vi "Automatic Extruder LabVIEW Program.vi"() -> ()   [LabVIEW 2022 SP3]
doc: "This VI allows to perform a single run pumping mode : the pump run continuously until the user decide to stop, reverse or pause it."
uses:
  <vilib>/Utility/error.llb/DialogType.ctl
  <vilib>/ptbypt/NI_PtbyPt.lvlib
panel:
  out "?":string
  out "Tank 4":dbl(slide) scale=0.0..1.0
  out "Tank 3":dbl(slide) scale=0.0..1000.0
  in  "Volume":string(combo)
  out "?":string
  out "Firmware Version :  2":string
  out "Extrusions Completed":i32
  out "Firmware Version :":string
  in  "Baud Rate (19200)":u32(ring)=19200 items=["19200"=19200, "9600"=9600, "2400"=2400, "1200"=1200, "300"=300]
  in  "Extrusions To Preform":i32
  in  "Master Pump Address":i32 format="%0#.0f"
  in  "Secondary Pump Resource":refnum<visa-resource-name>="COM4"
  in  "Master Pump VISA Resource":refnum<visa-resource-name>="COM3"
  in  "Secondary Pump Address":i32=1 format="%0#.0f"
  out "Tank 2":dbl(slide) scale=0.0..1000.0
  out "x+y":i32
  out "Tank":dbl(slide) scale=0.0..1.0
  in  "PAUSE 2":bool
  in  "PAUSE":bool
  in  "RUN":bool
  in  "STOP":bool
  in  "Audible Alarms":bool=TRUE
  in  "Flow rate":dbl=0.5 format="%.3f"
  in  "Units":i32(ring) items=["microlitters per minute (µL/min)", "microlitters per hour (µL/hr)", "milliliters per minute (mL/min)", "milliliters per hour (mL/hr)"]
  in  "Initial Direction":u16(ring) items=["Infuse", "Withdraw"]
  in  "Syringe Inside Diameter \nIf diameter is greater than 14.00 mm : Volume units are mL\nIf diameter is less than 14.00 mm : Volume units are µL":dbl=20.0 min=1.0 max=50.0 step=1.0
  out "Status":T1
  # "Configuration Settings"
  # "Master Pump Status"
  # "Volume"
  # "mm"
  # "Pump Control"
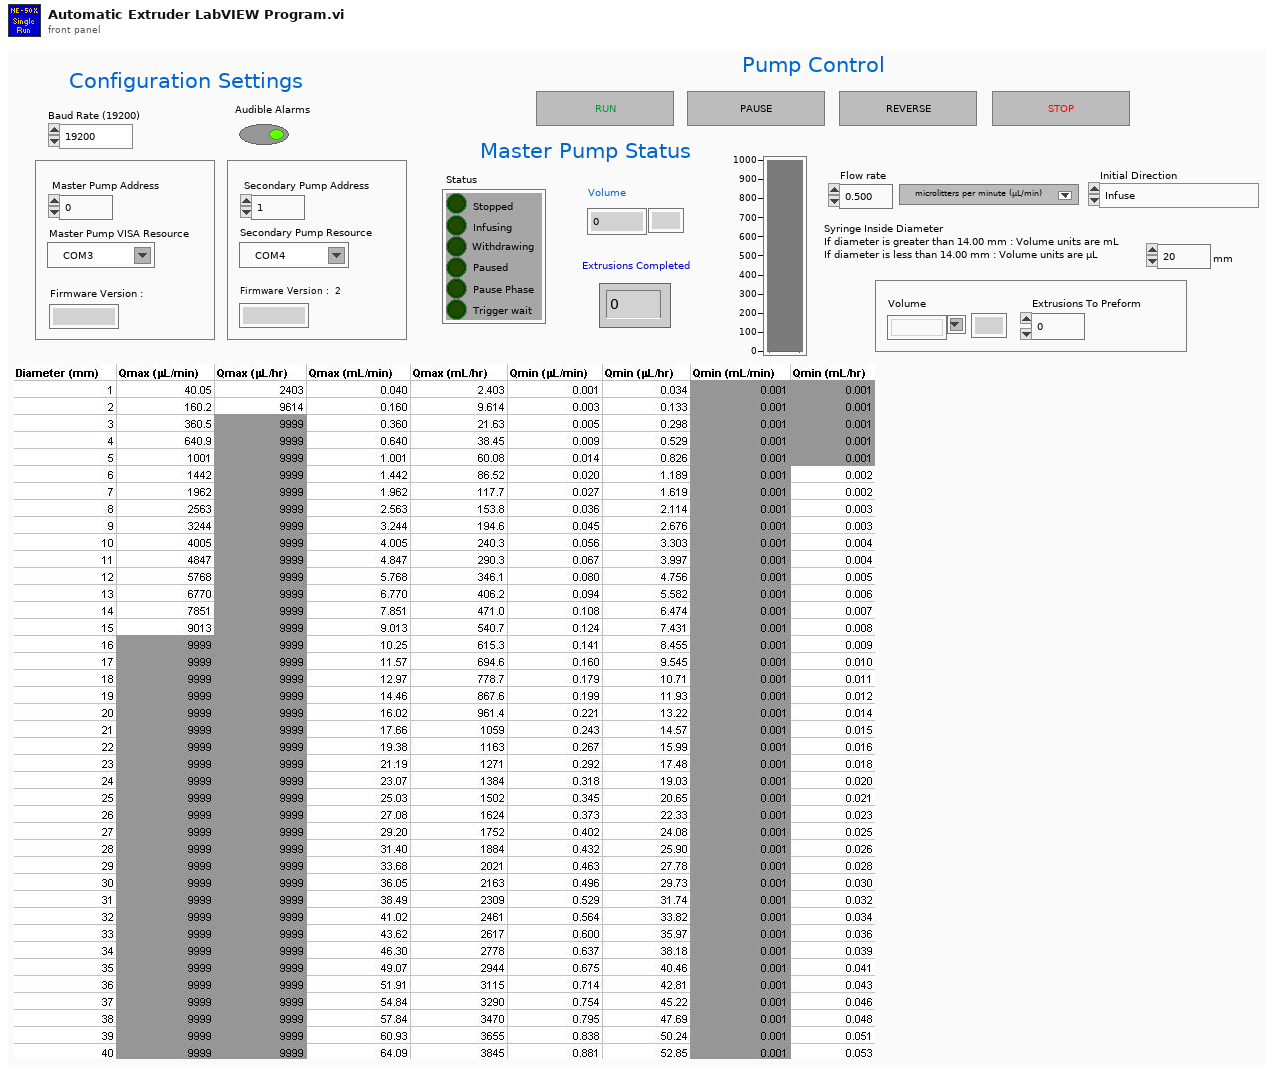
[diagram p1: front panel]
types:
  T1 = cluster{"Stopped":bool, "Infusing":bool, "Withdrawing":bool, "Paused":bool, "Pause Phase":bool, "Trigger wait":bool}
  T2 = typedef "DialogType.ctl" = u16
  T3 = cluster{"0=off\n1=on":u16, "Numbers of beeps\n0=continuously":dbl}
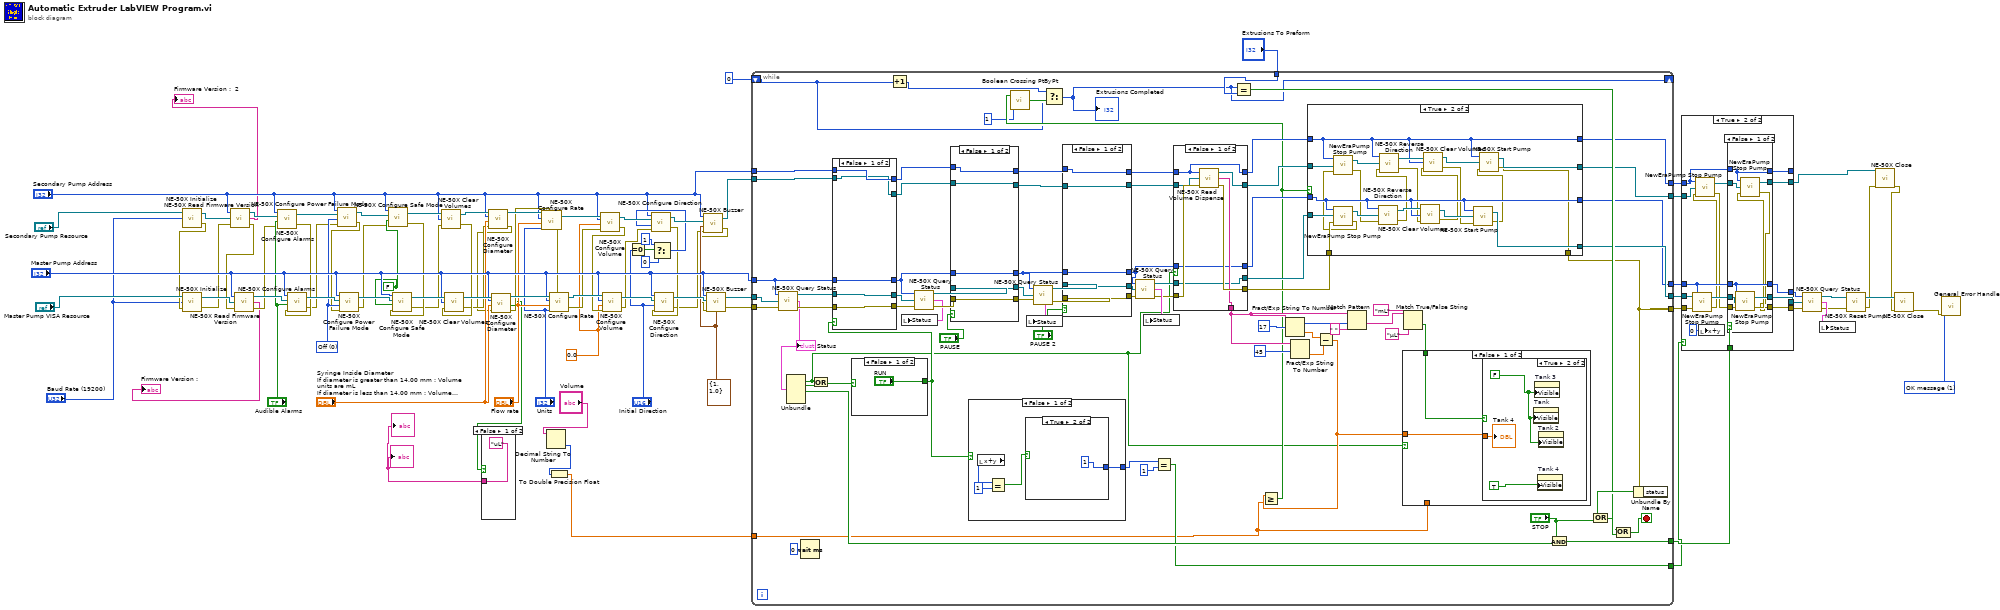
[diagram p0: block diagram]
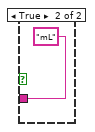
[diagram p2: hidden frame]
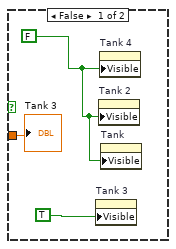
[diagram p5: hidden frame]
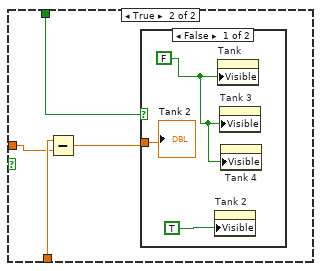
[diagram p6: hidden frame]
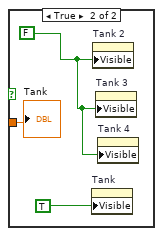
[diagram p7: hidden frame]
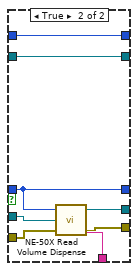
[diagram p8: hidden frame]
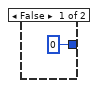
[diagram p10: hidden frame]
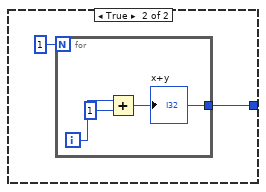
[diagram p11: hidden frame]
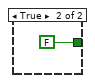
[diagram p12: hidden frame]
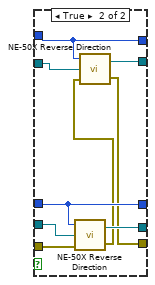
[diagram p13: hidden frame]
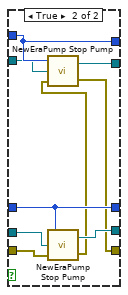
[diagram p14: hidden frame]
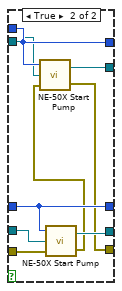
[diagram p15: hidden frame]
diagram:
  w8 = 0.0
  w70 = T2 1 items=["no dialog", "OK message", "continue or stop message", "OK message + warnings", "continue/stop + warnings"] ("type of dialog (OK msg:1)")
  w52 = FALSE ("0 = Basic")
  w51 = u16 0 items=["Off", "On"] ("0 = Disabled")
  w47 = T3 {"0=off\n1=on"=1, "Numbers of beeps\n0=continuously"=1.0} ("Buzzer")
  n1 = call <instrlib>:"NE-50X Initialize.vi"("Baud Rate (19200)"="Baud Rate (19200)", "VISA resource name"="Secondary Pump Resource") -> ("error out"=w40:errorcluster, "VISA resource name out"=w62:refnum<visa-resource-name>)  [unwired: 1 in]
  n2 = call <instrlib>:"NE-50X Initialize.vi"("error in (no error)"=w40, "Baud Rate (19200)"="Baud Rate (19200)", "VISA resource name"="Master Pump VISA Resource") -> ("error out"=w39:errorcluster, "VISA resource name out"=w78:refnum<visa-resource-name>)
  n3 = call <instrlib>:"NE-50X Read Firmware Version.vi"("error in (no error)"=w39, "VISA resource name"=w62, "Address (0)"="Secondary Pump Address") -> ("error out"=w38:errorcluster, "Version"=→"Firmware Version :  2":string, "VISA resource name out"=w61:refnum<visa-resource-name>)
  n4 = call <instrlib>:"NE-50X Read Firmware Version.vi"("error in (no error)"=w38, "VISA resource name"=w78, "Address (0)"="Master Pump Address") -> ("error out"=w37:errorcluster, "Version"=→"Firmware Version :":string, "VISA resource name out"=w79:refnum<visa-resource-name>)
  n5 = call <instrlib>:"NE-50X Configure Alarms.vi"("error in (no error)"=w37, "Audible Alarms"="Audible Alarms", "VISA resource name"=w61, "Address (0)"="Secondary Pump Address") -> ("error out"=w36:errorcluster, "VISA resource name out"=w60:refnum<visa-resource-name>)
  n6 = call <instrlib>:"NE-50X Configure Alarms.vi"("error in (no error)"=w36, "Audible Alarms"="Audible Alarms", "VISA resource name"=w79, "Address (0)"="Master Pump Address") -> ("error out"=w35:errorcluster, "VISA resource name out"=w80:refnum<visa-resource-name>)
  n7 = call <instrlib>:"NE-50X Configure Power Failure Mode.vi"("error in (no error)"=w35, "Power Failure Mode"=w51, "VISA resource name"=w60, "Address (0)"="Secondary Pump Address") -> ("error out"=w34:errorcluster, "VISA resource name out"=w59:refnum<visa-resource-name>)
  n8 = call <instrlib>:"NE-50X Configure Power Failure Mode.vi"("error in (no error)"=w34, "Power Failure Mode"=w51, "VISA resource name"=w80, "Address (0)"="Master Pump Address") -> ("error out"=w33:errorcluster, "VISA resource name out"=w81:refnum<visa-resource-name>)
  n9 = call <instrlib>:"NE-50X Configure Safe Mode.vi"("error in (no error)"=w33, "Safe Mode"=w52, "VISA resource name"=w59, "Address (0)"="Secondary Pump Address") -> ("error out"=w32:errorcluster, "VISA resource name out"=w58:refnum<visa-resource-name>)
  n10 = call <instrlib>:"NE-50X Configure Safe Mode.vi"("error in (no error)"=w32, "Safe Mode"=w52, "VISA resource name"=w81, "Address (0)"="Master Pump Address") -> ("error out"=w31:errorcluster, "VISA resource name out"=w69:refnum<visa-resource-name>)
  n11 = call <instrlib>:"NE-50X Clear Volumes.vi"("error in (no error)"=w31, "Address (0)"="Secondary Pump Address", "VISA resource name"=w58) -> ("error out"=w30:errorcluster, "VISA resource name out"=w57:refnum<visa-resource-name>)
  n12 = call <instrlib>:"NE-50X Clear Volumes.vi"("error in (no error)"=w30, "Address (0)"="Master Pump Address", "VISA resource name"=w69) -> ("error out"=w29:errorcluster, "VISA resource name out"=w66:refnum<visa-resource-name>)
  n13 = call <instrlib>:"NE-50X Configure Diameter.vi"("error in (no error)"=w29, "Diameter (19.58 mm)"="Syringe Inside Diameter \nIf diameter is greater than 14.00 mm : Volume units are mL\nIf diameter is less than 14.00 mm : Volume units are µL", "Address (0)"="Secondary Pump Address", "VISA resource name"=w57) -> ("error out"=w28:errorcluster, "VISA resource name out"=w56:refnum<visa-resource-name>)  [unwired: 1 in, 1 out]
  n14 = call <instrlib>:"NE-50X Configure Diameter.vi"("error in (no error)"=w28, "Diameter (19.58 mm)"="Syringe Inside Diameter \nIf diameter is greater than 14.00 mm : Volume units are mL\nIf diameter is less than 14.00 mm : Volume units are µL", "Address (0)"="Master Pump Address", "VISA resource name"=w66) -> ("error out"=w27:errorcluster, "Volume units"=w10:bool, "VISA resource name out"=w67:refnum<visa-resource-name>)  [unwired: 1 in]
  n15 = case shown="False" w10 {
    tunnel: ["uL" "mL"] -> w1
    frame False {
    }
    frame True {
    }
  }
  "?" <- w1
  "?" <- w1
  n16 = call <instrlib>:"NE-50X Configure Rate.vi"("VISA resource name"=w56, "Address (0)"="Secondary Pump Address", "Flow"="Flow rate", "Units"="Units", "error in (no error)"=w27) -> ("VISA resource name out"=w55:refnum<visa-resource-name>, "error out"=w26:errorcluster)
  n17 = Decimal String To Number(string="Volume") -> (number=w6:i32)  [unwired: 2 in, 1 out]
  n18 = call <instrlib>:"NE-50X Configure Rate.vi"("VISA resource name"=w67, "Address (0)"="Master Pump Address", "Flow"="Flow rate", "Units"="Units", "error in (no error)"=w26) -> ("VISA resource name out"=w68:refnum<visa-resource-name>, "error out"=w25:errorcluster)
  n19 = To Double Precision Float(number=w6) -> (double precision float=w5:dbl)
  n20 = call <instrlib>:"NE-50X Configure Volume.vi"("error in (no error)"=w25, "Volume"=w8, "Address (0)"="Secondary Pump Address", "VISA resource name"=w55) -> ("error out"=w24:errorcluster, "VISA resource name out"=w54:refnum<visa-resource-name>)
  n21 = call <instrlib>:"NE-50X Configure Volume.vi"("error in (no error)"=w24, "Volume"=w8, "Address (0)"="Master Pump Address", "VISA resource name"=w68) -> ("error out"=w23:errorcluster, "VISA resource name out"=w82:refnum<visa-resource-name>)
  n22 = Equal To 0?(x="Initial Direction") -> (x = 0?=w45:bool)
  n23 = Select(t=u16 1, s=w45, f=u16 0) -> (s? t:f=w41:u16)
  n24 = call <instrlib>:"NE-50X Configure Direction.vi"("error in (no error)"=w23, "Direction"=w41, "VISA resource name"=w54, "Address (0)"="Secondary Pump Address") -> ("error out"=w22:errorcluster, "VISA resource name out"=w53:refnum<visa-resource-name>)
  n25 = call <instrlib>:"NE-50X Configure Direction.vi"("error in (no error)"=w22, "Direction"="Initial Direction", "VISA resource name"=w82, "Address (0)"="Master Pump Address") -> ("error out"=w21:errorcluster, "VISA resource name out"=w83:refnum<visa-resource-name>)
  n26 = call <instrlib>:"NE-50X Buzzer.vi"("error in (no error)"=w21, "Buzzer"=w47, "VISA resource name"=w53, "Address (0)"="Secondary Pump Address") -> ("error out"=w20:errorcluster, "VISA resource name out"=w18:refnum<visa-resource-name>)
  n27 = call <instrlib>:"NE-50X Buzzer.vi"("error in (no error)"=w20, "Buzzer"=w47, "VISA resource name"=w83, "Address (0)"="Master Pump Address") -> ("error out"=w86:errorcluster, "VISA resource name out"=w85:refnum<visa-resource-name>)
  n28 = while {
    tunnel: w85 -> [w149]
    tunnel: w86 -> [w170]
    tunnel: [w118] -> w77
    tunnel: [w119] -> w84
    tunnel: "Master Pump Address" -> [w148]
    tunnel: [w115] -> w76
    tunnel: [w141] -> w74
    tunnel: [w137] -> w72
    tunnel: "Secondary Pump Address" -> [w131]
    tunnel: w18 -> [w129]
    tunnel: [w117] -> w16
    tunnel: [w114] -> w17
    tunnel: w5 -> [w93]
    tunnel: "Extrusions To Preform" -> [w116]
    shift-right: [w97] -> _
    shift-left: 0 -> [w98]
    stop <- w122 stop-if-true
    n29 = call <instrlib>:"NE-50X Query Status.vi"("error in (no error)"=w170, "VISA resource name"=w149, "Address (0)"=w148) -> ("error out"=w167:errorcluster, "Status"=w161:T1, "VISA resource name out"=w168:refnum<visa-resource-name>)
    "Status" <- w161
    n30 = Unbundle(w161) -> ("Infusing"=w94:bool, "Withdrawing"=w160:bool, "Paused"=w142:bool)  [unwired: 3 out]
    n31 = Wait (ms)(milliseconds to wait=u32 0) -> ()  [unwired: 1 out]
    n32 = Or(x=w94, y=w160) -> (x .or. y?=w159:bool)
    n33 = case shown="False" w159 {
      tunnel: ["RUN" FALSE ("RUN")] -> w138
      frame False {
      }
      frame True {
      }
    }
    n34 = case shown="False" w138 {
      tunnel: w148 -> [w277 w283]
      tunnel: [w276 w286] -> w145
      tunnel: [w275 w278] -> w158
      tunnel: [w277 w283] -> w147
      tunnel: w168 -> [w276 w284]
      tunnel: w167 -> [w275 w285]
      tunnel: w131 -> [w274 w282]
      tunnel: [w274 w282] -> w130
      tunnel: w129 -> [w273 w281]
      tunnel: [w273 w280] -> w128
      frame False {
      }
      frame True {
        n35 = call <instrlib>:"NE-50X Start Pump.vi"("error in (no error)"=w285, "VISA resource name"=w284, "Address (0)"=w283) -> ("error out"=w279:errorcluster, "VISA resource name out"=w286:refnum<visa-resource-name>)
        n36 = call <instrlib>:"NE-50X Start Pump.vi"("error in (no error)"=w279, "VISA resource name"=w281, "Address (0)"=w282) -> ("error out"=w278:errorcluster, "VISA resource name out"=w280:refnum<visa-resource-name>)
      }
    }
    n37 = Increment(x=w98) -> (x+1=w99:i32)
    n38 = call <instrlib>:"NE-50X Query Status.vi"("error in (no error)"=w158, "VISA resource name"=w145, "Address (0)"=w147) -> ("error out"=w157:errorcluster, "Status"=w152:T1, "VISA resource name out"=w156:refnum<visa-resource-name>)
    n39 = local write "Status"(w152) -> ()
    n40 = case shown="False" "PAUSE" {
      tunnel: w147 -> [w263 w269]
      tunnel: w156 -> [w261 w270]
      tunnel: w157 -> [w262 w272]
      tunnel: [w262 w264] -> w155
      tunnel: [w261 w271] -> w146
      tunnel: [w263 w269] -> w126
      tunnel: w130 -> [w260 w268]
      tunnel: [w260 w268] -> w125
      tunnel: w128 -> [w259 w267]
      tunnel: [w259 w266] -> w127
      frame False {
      }
      frame True {
        n41 = call <instrlib>:"NewEraPump Stop Pump.vi"("error in (no error)"=w272, "VISA resource name"=w270, "Address (0)"=w269) -> ("error out"=w265:errorcluster, "VISA resource name out"=w271:refnum<visa-resource-name>)
        n42 = call <instrlib>:"NewEraPump Stop Pump.vi"("error in (no error)"=w265, "VISA resource name"=w267, "Address (0)"=w268) -> ("error out"=w264:errorcluster, "VISA resource name out"=w266:refnum<visa-resource-name>)
      }
    }
    n43 = case shown="False" w138 {
      tunnel: [w232 w238] -> w140
      frame False {
        n44 = local read "x+y"() -> (w235:i32)
        n45 = Equal?(x=w235, y=1) -> (x = y?=w233:bool)
        n46 = case shown="True" w233 {
          tunnel: [0 1] -> w232
          frame False {
          }
          frame True {
          }
        }
      }
      frame True {
        n47 = for {
          N: 1 -> [_]
          tunnel: [w240] -> w238
          i -> [w242]
          n48 = Add(x=w242, y=1) -> (x+y=w240:i32)
          "x+y" <- w240
        }
      }
    }
    n49 = call <instrlib>:"NE-50X Query Status.vi"("error in (no error)"=w155, "VISA resource name"=w146, "Address (0)"=w126) -> ("error out"=w153:errorcluster, "Status"=w151:T1, "VISA resource name out"=w154:refnum<visa-resource-name>)
    n50 = local write "Status"(w151) -> ()
    n51 = case shown="False" "PAUSE 2" {
      tunnel: w154 -> [w249 w255]
      tunnel: w126 -> [w247 w256]
      tunnel: [w249 w258] -> w120
      tunnel: [w248 w250] -> w121
      tunnel: w153 -> [w248 w257]
      tunnel: [w247 w256] -> w108
      tunnel: w125 -> [w246 w254]
      tunnel: [w246 w254] -> w112
      tunnel: w127 -> [w245 w253]
      tunnel: [w245 w252] -> w111
      frame False {
      }
      frame True {
        n52 = call <instrlib>:"NE-50X Reverse Direction.vi"("error in (no error)"=w257, "VISA resource name"=w255, "Address (0)"=w256) -> ("error out"=w251:errorcluster, "VISA resource name out"=w258:refnum<visa-resource-name>)
        n53 = call <instrlib>:"NE-50X Reverse Direction.vi"("error in (no error)"=w251, "VISA resource name"=w253, "Address (0)"=w254) -> ("error out"=w250:errorcluster, "VISA resource name out"=w252:refnum<visa-resource-name>)
      }
    }
    n54 = call <instrlib>:"NE-50X Query Status.vi"("error in (no error)"=w121, "VISA resource name"=w120, "Address (0)"=w108) -> ("error out"=w104:errorcluster, "Status"=w150:T1, "VISA resource name out"=w106:refnum<visa-resource-name>)
    n55 = local write "Status"(w150) -> ()
    n56 = Equal?(x=w140, y=1) -> (x = y?=w137:bool)
    n57 = case shown="False" w94 {
      tunnel: [w192 w205] -> w113
      tunnel: w112 -> [w193 w204]
      tunnel: w111 -> [w195 w203]
      tunnel: [w193 w204] -> w110
      tunnel: [w194 w203] -> w109
      tunnel: w108 -> [w191 w202]
      tunnel: [w191 w202] -> w107
      tunnel: w106 -> [w190 w201]
      tunnel: [w190 w200] -> w105
      tunnel: w104 -> [w197 w199]
      tunnel: [w196 w198] -> w103
      frame False {
        n58 = call <instrlib>:"NE-50X Read Volume Dispense.vi"("error in (no error)"=w197, "VISA resource name"=w195, "Address (0)"=w193) -> ("error out"=w196:errorcluster, "Volume Dispense"=w192:string, "VISA resource name out"=w194:refnum<visa-resource-name>)
      }
      frame True {
        n59 = call <instrlib>:"NE-50X Read Volume Dispense.vi"("error in (no error)"=w199, "VISA resource name"=w201, "Address (0)"=w202) -> ("error out"=w198:errorcluster, "Volume Dispense"=w205:string, "VISA resource name out"=w200:refnum<visa-resource-name>)
      }
    }
    n60 = Fract/Exp String To Number(string=w113, offset=17) -> (offset past number=w135:i32, number=w163:dbl)  [unwired: 2 in]
    n61 = Fract/Exp String To Number(string=w113, offset=45) -> (number=w162:dbl)  [unwired: 2 in, 1 out]
    n62 = Subtract(x=w163, y=w162) -> (x-y=w96:dbl)
    n63 = Greater Or Equal?(x=w96, y=w93) -> (x >= y?=w101:bool)
    n64 = call <vilib>:"Boolean Crossing PtByPt.vi"("direction"=1, "input"=w101) -> ("crossing"=w102:bool)  [unwired: 1 in]
    n65 = Select(t=w99, s=w102, f=w98) -> (s? t:f=w97:i32)
    "Extrusions Completed" <- w97
    n66 = Equal?(x=w97, y=w116) -> (x = y?=w124:bool)
    n67 = case shown="True" w101 {
      tunnel: [w206 w211] -> w119
      tunnel: [w207 w220] -> w118
      tunnel: [w209 w224] -> w117
      tunnel: w110 -> [w210 w229]
      tunnel: [w210 w229] -> w114
      tunnel: w107 -> [w208 w228]
      tunnel: [w208 w228] -> w115
      tunnel: w109 -> [w209 w227]
      tunnel: w105 -> [w207 w223]
      tunnel: w103 -> [w206 w219]
      frame False {
      }
      frame True {
        n68 = call <instrlib>:"NewEraPump Stop Pump.vi"("error in (no error)"=w219, "VISA resource name"=w223, "Address (0)"=w228) -> ("error out"=w218:errorcluster, "VISA resource name out"=w222:refnum<visa-resource-name>)
        n69 = call <instrlib>:"NewEraPump Stop Pump.vi"("error in (no error)"=w218, "VISA resource name"=w227, "Address (0)"=w229) -> ("error out"=w217:errorcluster, "VISA resource name out"=w226:refnum<visa-resource-name>)
        n70 = call <instrlib>:"NE-50X Reverse Direction.vi"("error in (no error)"=w217, "VISA resource name"=w222, "Address (0)"=w228) -> ("error out"=w216:errorcluster, "VISA resource name out"=w231:refnum<visa-resource-name>)
        n71 = call <instrlib>:"NE-50X Reverse Direction.vi"("error in (no error)"=w216, "VISA resource name"=w226, "Address (0)"=w229) -> ("error out"=w215:errorcluster, "VISA resource name out"=w230:refnum<visa-resource-name>)
        n72 = call <instrlib>:"NE-50X Clear Volumes.vi"("error in (no error)"=w215, "Address (0)"=w228, "VISA resource name"=w231) -> ("error out"=w214:errorcluster, "VISA resource name out"=w221:refnum<visa-resource-name>)
        n73 = call <instrlib>:"NE-50X Clear Volumes.vi"("error in (no error)"=w214, "Address (0)"=w229, "VISA resource name"=w230) -> ("error out"=w213:errorcluster, "VISA resource name out"=w225:refnum<visa-resource-name>)
        n74 = call <instrlib>:"NE-50X Start Pump.vi"("error in (no error)"=w213, "VISA resource name"=w221, "Address (0)"=w228) -> ("error out"=w212:errorcluster, "VISA resource name out"=w220:refnum<visa-resource-name>)
        n75 = call <instrlib>:"NE-50X Start Pump.vi"("error in (no error)"=w212, "VISA resource name"=w225, "Address (0)"=w229) -> ("error out"=w211:errorcluster, "VISA resource name out"=w224:refnum<visa-resource-name>)
      }
    }
    n76 = Match Pattern(string=w113, regular expression=" ", offset (0)=w135) -> (after substring=w132:string)  [unwired: 3 out]
    n77 = Match True/False String(2:"µL" ("false string"), 3:"mL" ("true string"), 4:w132) -> (0:w95:bool)  [unwired: 1 out]
    n78 = case shown="False" w94 {
      tunnel: w96 -> [w172 w181]
      tunnel: w95 -> [w173 w183]
      tunnel: w93 -> [_ w182]
      frame False {
        n79 = case shown="True" w173 {
          tunnel: w172 -> [w176 w179]
          frame False {
            w174 = FALSE ("Visible")
            n80 = property on="Tank 3" class="Slide (strict)"("Visible"=TRUE) -> ()  [unwired: 2 in, 2 out]
            n81 = property on="Tank 2" class="Slide (strict)"("Visible"=w174) -> ()  [unwired: 2 in, 2 out]
            n82 = property on="Tank 4" class="Slide (strict)"("Visible"=w174) -> ()  [unwired: 2 in, 2 out]
            n83 = property on="Tank" class="Slide (strict)"("Visible"=w174) -> ()  [unwired: 2 in, 2 out]
            "Tank 3" <- w176
          }
          frame True {
            w177 = FALSE
            n84 = property on="Tank" class="Slide (strict)"("Visible"=w177) -> ()  [unwired: 2 in, 2 out]
            n85 = property on="Tank 3" class="Slide (strict)"("Visible"=w177) -> ()  [unwired: 2 in, 2 out]
            n86 = property on="Tank 4" class="Slide (strict)"("Visible"=TRUE) -> ()  [unwired: 2 in, 2 out]
            n87 = property on="Tank 2" class="Slide (strict)"("Visible"=w177) -> ()  [unwired: 2 in, 2 out]
            "Tank 4" <- w179
          }
        }
      }
      frame True {
        n88 = Subtract(x=w182, y=w181) -> (x-y=w180:dbl)
        n89 = case shown="False" w183 {
          tunnel: w180 -> [w186 w189]
          frame False {
            w184 = FALSE ("Visible")
            n90 = property on="Tank 2" class="Slide (strict)"("Visible"=TRUE) -> ()  [unwired: 2 in, 2 out]
            n91 = property on="Tank" class="Slide (strict)"("Visible"=w184) -> ()  [unwired: 2 in, 2 out]
            n92 = property on="Tank 3" class="Slide (strict)"("Visible"=w184) -> ()  [unwired: 2 in, 2 out]
            n93 = property on="Tank 4" class="Slide (strict)"("Visible"=w184) -> ()  [unwired: 2 in, 2 out]
            "Tank 2" <- w186
          }
          frame True {
            w187 = FALSE
            n94 = property on="Tank" class="Slide (strict)"("Visible"=TRUE) -> ()  [unwired: 2 in, 2 out]
            n95 = property on="Tank 2" class="Slide (strict)"("Visible"=w187) -> ()  [unwired: 2 in, 2 out]
            n96 = property on="Tank 3" class="Slide (strict)"("Visible"=w187) -> ()  [unwired: 2 in, 2 out]
            n97 = property on="Tank 4" class="Slide (strict)"("Visible"=w187) -> ()  [unwired: 2 in, 2 out]
            "Tank" <- w189
          }
        }
      }
    }
    n98 = And(x="STOP", y=w142) -> (x .and. y?=w141:bool)
    n99 = Unbundle By Name(w119) -> ("status"=w144:bool)
    n100 = Compound Arithmetic op=OR(w144, "STOP") -> (w123:bool)
    n101 = Compound Arithmetic op=OR(w123, w124) -> (w122:bool)
  }
  n102 = case shown="True" w72 {
    tunnel: [w289 w307] -> w89
    tunnel: w84 -> [w289 w306]
    tunnel: w77 -> [w290 w305]
    tunnel: w76 -> [w291 w304]
    tunnel: [w290 w303] -> w75
    tunnel: w74 -> [_ w302]
    tunnel: [w291 w301] -> w73
    tunnel: w17 -> [w288 w295]
    tunnel: w16 -> [w287 w298]
    tunnel: [w287 w296] -> w3
    tunnel: [w288 w294] -> _
    frame False {
    }
    frame True {
      n103 = call <instrlib>:"NewEraPump Stop Pump.vi"("error in (no error)"=w306, "VISA resource name"=w305, "Address (0)"=w304) -> ("error out"=w293:errorcluster, "VISA resource name out"=w300:refnum<visa-resource-name>)
      n104 = call <instrlib>:"NewEraPump Stop Pump.vi"("error in (no error)"=w293, "VISA resource name"=w298, "Address (0)"=w295) -> ("error out"=w292:errorcluster, "VISA resource name out"=w297:refnum<visa-resource-name>)
      n105 = local write "x+y"(0 ("x+y")) -> ()
      n106 = case shown="False" w302 {
        tunnel: w292 -> [w316 w321]
        tunnel: [w308 w321] -> w307
        tunnel: w304 -> [w313 w319]
        tunnel: [w315 w320] -> w303
        tunnel: w300 -> [w314 w320]
        tunnel: [w313 w319] -> w301
        tunnel: w297 -> [w312 w317]
        tunnel: [w311 w317] -> w296
        tunnel: w295 -> [w310 w318]
        tunnel: [w310 w318] -> w294
        frame False {
          n107 = call <instrlib>:"NewEraPump Stop Pump.vi"("error in (no error)"=w316, "VISA resource name"=w314, "Address (0)"=w313) -> ("error out"=w309:errorcluster, "VISA resource name out"=w315:refnum<visa-resource-name>)
          n108 = call <instrlib>:"NewEraPump Stop Pump.vi"("error in (no error)"=w309, "VISA resource name"=w312, "Address (0)"=w310) -> ("error out"=w308:errorcluster, "VISA resource name out"=w311:refnum<visa-resource-name>)
        }
        frame True {
        }
      }
    }
  }
  n109 = call <instrlib>:"NE-50X Query Status.vi"("error in (no error)"=w89, "VISA resource name"=w75, "Address (0)"=w73) -> ("error out"=w2:errorcluster, "Status"=w87:T1, "VISA resource name out"=w88:refnum<visa-resource-name>)
  n110 = local write "Status"(w87) -> ()
  n111 = call <instrlib>:"NE-50X Reset Pump.vi"("error in (no error)"=w2, "VISA resource name"=w88) -> ("error out"=w15:errorcluster, "VISA resource name out"=w90:refnum<visa-resource-name>)
  n112 = call <instrlib>:"NE-50X Close.vi"("VISA resource name"=w3, "error in (no error)"=w15) -> ("error out"=w14:errorcluster)  [unwired: 13 in]
  n113 = call <instrlib>:"NE-50X Close.vi"("VISA resource name"=w90, "error in (no error)"=w14) -> ("error out"=w71:errorcluster)  [unwired: 13 in]
  n114 = call <vilib>:"General Error Handler.vi"("type of dialog (OK msg:1)"=w70, "error in (no error)"=w71) -> ()  [unwired: 9 in, 5 out]
